vi "hse-config-ini_WriteKey.vi"(6 "Value":string, 8 "error in (no error)":errorcluster, 9 "Key":string, 10 "Section":string, 11 "hse-config-ini in":refnum<class "hse-config-ini.lvclass">) -> (0 "error out":errorcluster, 3 "hse-config-ini out":refnum<class "hse-config-ini.lvclass">)   [LabVIEW 2020, in "hse-config-ini.lvclass"]
doc: "____\nHAMPEL SOFTWARE ENGINEERING v3.8.0 (2023-12-18 14:41)"
uses:
  hse-config-ini.lvclass
  hse-config-ini.lvclass/hse-config-ini.ctl
  <vilib>/Utility/config.llb/NI_LVConfig.lvlib
  <vilib>/Utility/config.llb/Write Key (String).vi
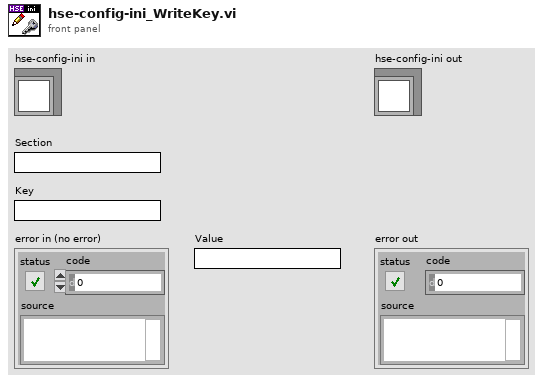
[diagram p1: front panel]
types:
  T1 = typedef "NI_LVConfig.lvlib/Config Data RefNum.ctl" = refnum<k1>
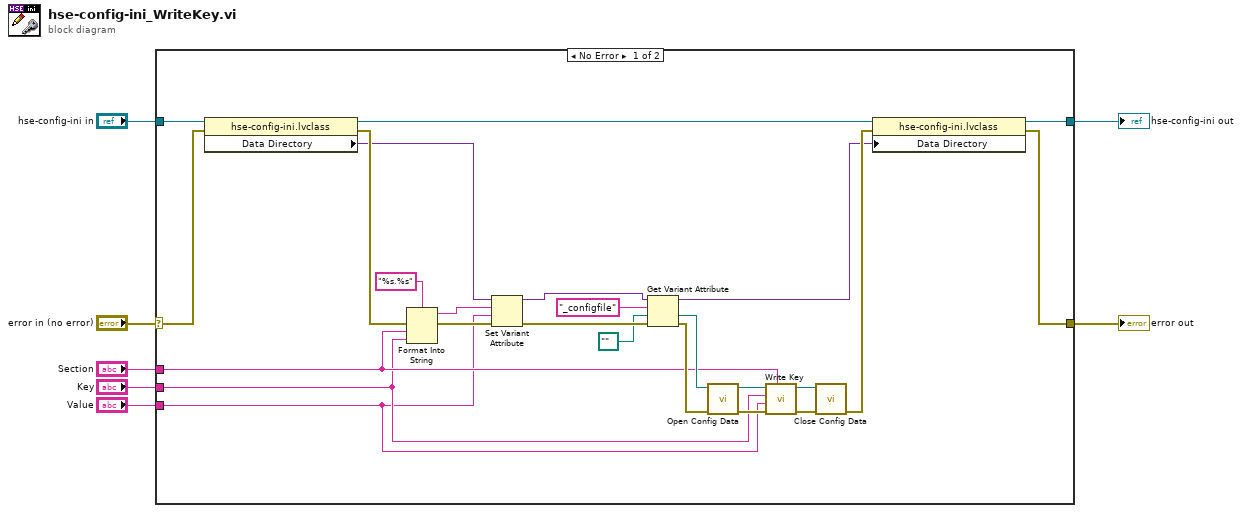
[diagram p0: block diagram]
diagram:
  n1 = case shown="No Error" "error in (no error)" {
    selector: "error in (no error)" -> [w27 w33]
    tunnel: [w12 w33] -> w7
    tunnel: "Key" -> [w9 _]
    tunnel: "Section" -> [w10 _]
    tunnel: [w20 w34] -> w3
    tunnel: "hse-config-ini in" -> [w24 w34]
    tunnel: "Value" -> [w8 _]
    frame No Error {
      n2 = property class="hse-config-ini.lvclass"(reference=w24, error in=w27) -> (reference out=w25:refnum<class "hse-config-ini.lvclass">, error out=w28:errorcluster, "Data Directory"=w26:variant)
      n3 = Format Into String(format string="%s.%s", error in=w28, w10, w9) -> (resulting string=w23:string, error out=w29:errorcluster)  [unwired: 1 in]
      n4 = Set Variant Attribute(Variant=w26, name=w23, value=w8, error in=w29) -> (Variant out=w19:variant, error out=w32:errorcluster)  [unwired: 1 out]
      n5 = Get Variant Attribute(Variant=w19, name="_configfile", default value (empty Variant)=path "", error in=w32) -> (duplicate Variant=w18:variant, value=w11:path, error out=w17:errorcluster)  [unwired: 1 out]
      n6 = call <vilib>:"Open Config Data.vi"("error in (no error)"=w17, "configuration file path"=w11) -> ("error out"=w15:errorcluster, "refnum"=w16:T1)  [unwired: 7 in, 1 out]
      n7 = call-poly <vilib>:"Write Key.vi"("section"=w10, "error in (no error)"=w15, "value"=w8, "key"=w9, "refnum"=w16) -> ("error out"=w13:errorcluster, "refnum out"=w14:T1)  [unwired: 4 in, 1 out]
      n8 = call <vilib>:"Close Config Data.vi"("error in (no error)"=w13, "refnum"=w14) -> ("error out"=w31:errorcluster)  [unwired: 8 in, 1 out]
      n9 = property class="hse-config-ini.lvclass"(reference=w25, error in=w31, "Data Directory"=w18) -> (reference out=w20:refnum<class "hse-config-ini.lvclass">, error out=w12:errorcluster)
    }
    frame Error {
    }
  }
  "error out" <- w7
  "hse-config-ini out" <- w3
